vi "Data_Fit.vi"(6 "error in (no error)":errorcluster, 10 "Mass Flow (lbm/min) vs. Pressure Drop (inH2O) - Real Data":dbl[][](array[numeric]), 11 "total_dp_inh2o":dbl[](array[numeric])) -> (0 "Power - Sim":string, 1 "Amplitude - Sim":string, 2 "Power - Empirical":string, 3 "Amplitude - Empirical":string, 4 "error out":errorcluster)   [LabVIEW 2025]
uses:
  <vilib>/Analysis/NI_AALPro.lvlib
panel:
  # "Empirical Fit"
  # "P"
  # "="
  # "* X"
  # "drop"
  # "Simulator Fit"
  # "P"
  # "="
  # "* X"
  # "drop"
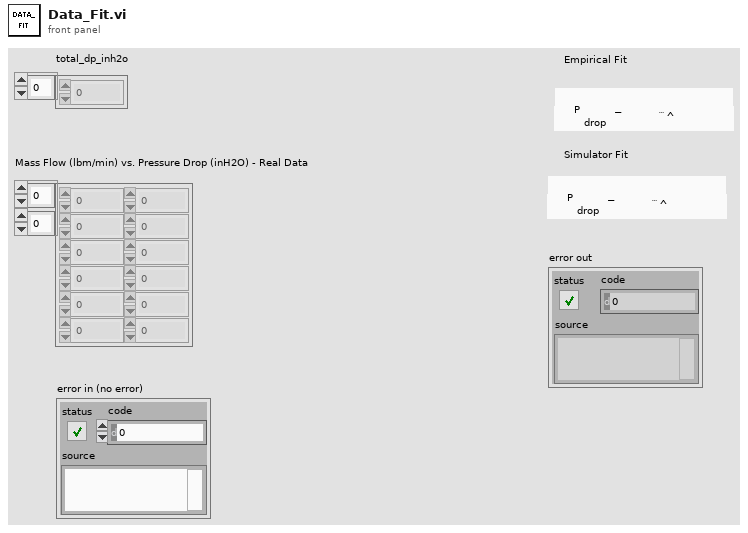
[diagram p1: front panel]
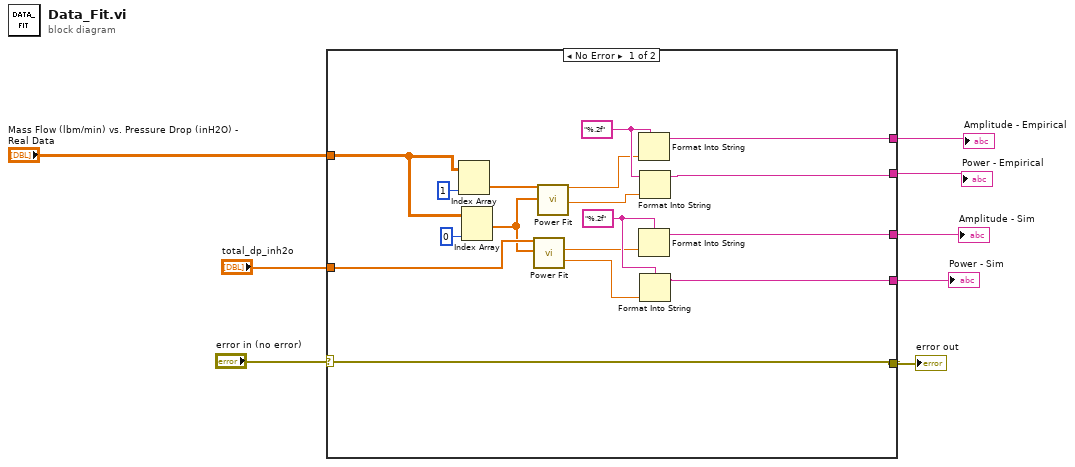
[diagram p0: block diagram]
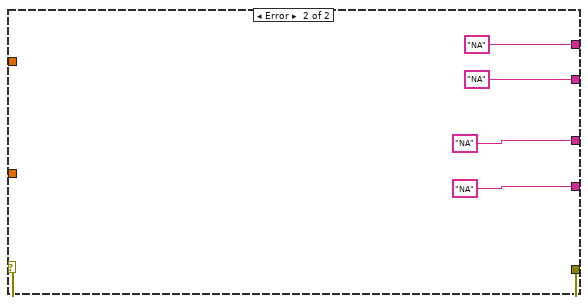
[diagram p2: hidden frame]
diagram:
  n1 = case shown="No Error" "error in (no error)" {
    selector: "error in (no error)" -> [w14 w30]
    tunnel: "Mass Flow (lbm/min) vs. Pressure Drop (inH2O) - Real Data" -> [w13 _]
    tunnel: "total_dp_inh2o" -> [w19 _]
    tunnel: [w14 w30] -> w5
    tunnel: [w12 "NA"] -> w4
    tunnel: [w11 "NA"] -> w3
    tunnel: [w10 "NA"] -> w1
    tunnel: [w9 "NA"] -> w2
    frame No Error {
      w25 = "%.2f" ("format string")
      w24 = "%.2f" ("format string")
      n2 = Index Array(array=w13, index (col)=1 ("disabled index (col)")) -> (element=w17:dbl[])  [unwired: 1 in]
      n3 = Index Array(array=w13, index (col)=0 ("disabled index (col)")) -> (element=w18:dbl[])  [unwired: 1 in]
      n4 = call <vilib>:"Power Fit.vi"("Y"=w19, "X"=w18) -> ("amplitude"=w20:dbl, "power"=w21:dbl)  [unwired: 8 in, 4 out]
      n5 = call <vilib>:"Power Fit.vi"("Y"=w17, "X"=w18) -> ("amplitude"=w23:dbl, "power"=w22:dbl)  [unwired: 8 in, 4 out]
      n6 = Format Into String(format string=w25, w23) -> (resulting string=w12:string)  [unwired: 2 in, 1 out]
      n7 = Format Into String(format string=w24, w20) -> (resulting string=w10:string)  [unwired: 2 in, 1 out]
      n8 = Format Into String(format string=w25, w22) -> (resulting string=w11:string)  [unwired: 2 in, 1 out]
      n9 = Format Into String(format string=w24, w21) -> (resulting string=w9:string)  [unwired: 2 in, 1 out]
    }
    frame Error {
    }
  }
  "error out" <- w5
  "Amplitude - Empirical" <- w4
  "Power - Empirical" <- w3
  "Power - Sim" <- w2
  "Amplitude - Sim" <- w1
